vi "Transfer.vi"(8 "file path":path, 9 "Input String":string, 10 "Account No.":string) -> (2 "Output":string)   [LabVIEW 2023]
uses:
  <vilib>/regexp/Match Regular Expression.xnode
panel:
  # "Input"
  # "Output"
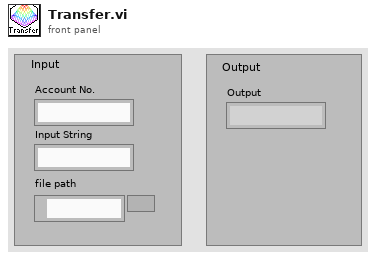
[diagram p1: front panel]
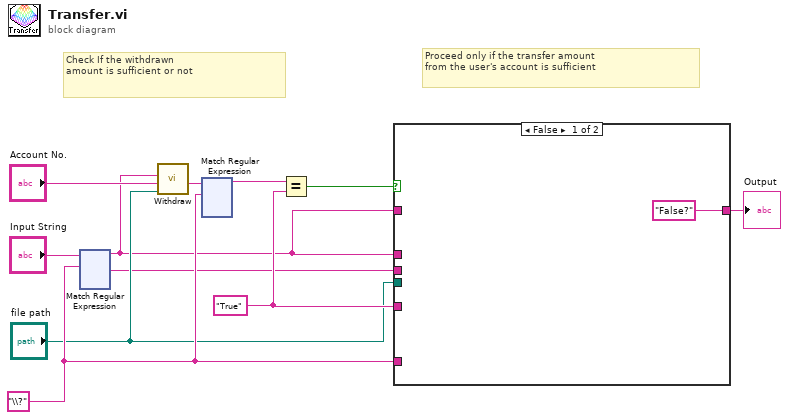
[diagram p0: block diagram]
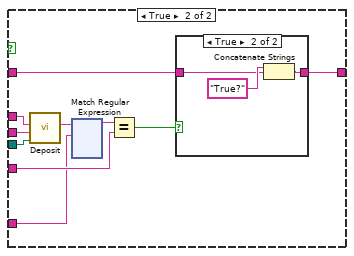
[diagram p2: hidden frame]
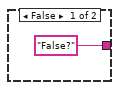
[diagram p3: hidden frame]
diagram:
  w6 = "True" ("y")
  w5 = "\\?" ("regular expression")
  # "Proceed only if the transfer amount \nfrom the user's account is sufficient"
  # "Check If the withdrawn \namount is sufficient or not"
  n1 = xnode ("Match Regular \nExpression")("input string"="Input String", "regular expression"=w5) -> ("before match"=w2:string, "after match"=w3:string)  [unwired: 4 in, 3 out]
  n2 = call "Withdraw.vi"("file path"="file path", "Account No."="Account No.", "Amount"=w2) -> ("Output"=w10:string)  [unwired: 8 in]
  n3 = xnode ("Match Regular \nExpression")("input string"=w10, "regular expression"=w5) -> ("before match"=w11:string)  [unwired: 4 in, 4 out]
  n4 = Equal?(x=w11, y=w6) -> (x = y?=w7:bool)
  n5 = case shown="False" w7 {
    tunnel: w6 -> [_ w20]
    tunnel: w5 -> [_ w19]
    tunnel: "file path" -> [_ w18]
    tunnel: w3 -> [_ w17]
    tunnel: w2 -> [_ w16]
    tunnel: w2 -> [_ w15]
    tunnel: ["False?" w13] -> w1
    frame False {
    }
    frame True {
      n6 = call "Deposit.vi"("file path"=w18, "Account No."=w17, "Amount"=w16) -> ("Output"=w22:string)  [unwired: 8 in]
      n7 = xnode ("Match Regular \nExpression")("input string"=w22, "regular expression"=w19) -> ("before match"=w21:string)  [unwired: 4 in, 4 out]
      n8 = Equal?(x=w21, y=w20) -> (x = y?=w14:bool)
      n9 = case shown="True" w14 {
        tunnel: w15 -> [_ w25]
        tunnel: ["False?" w24] -> w13
        frame False {
        }
        frame True {
          n10 = Concatenate Strings("True?" ("String"), w25) -> (w24:string)
        }
      }
    }
  }
  "Output" <- w1
